vi "规范时间戳.vi"(11 "字符串":string) -> (3 "result string":string)   [LabVIEW 2016, in "数据传输系统.lvlib"]
panel:
  out "输出 1":timestamp
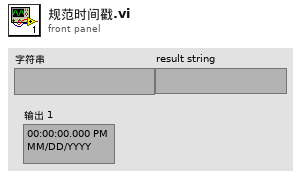
[diagram p1: front panel]
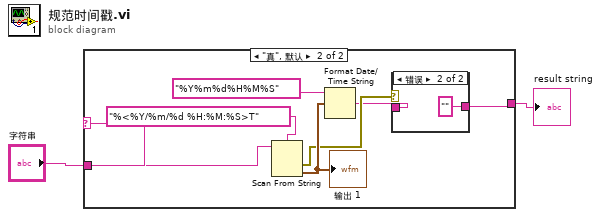
[diagram p0: block diagram]
diagram:
  n1 = case shown="\"真\", 默认" "字符串" {
    tunnel: "字符串" -> [w3 w10]
    tunnel: [w3 w4] -> w2
    frame "" {
    }
    frame "真", Default {
      n2 = Scan From String(format string="%<%Y/%m/%d %H:%M:%S>T" ("格式字符串"), input string=w10) -> (error out=w6:errorcluster, output 1=w9:timestamp)  [unwired: 3 in, 2 out]
      "输出 1" <- w9
      n3 = Format Date/Time String(time format string (%c)="%Y%m%d%H%M%S" ("时间格式字符串(%c)"), seconds (now)=w9) -> (date/time string=w5:string)  [unwired: 1 in]
      n4 = case shown="错误" w6 {
        tunnel: [w11 "" ("date/time string")] -> w4
        tunnel: w5 -> [w11 _]
        frame No Error {
        }
        frame Error {
        }
      }
    }
  }
  "result string" <- w2
